vi "Get Number of Layers (SubVI).vi"(4 "error IN":errorcluster, 5 "Layers Array":T1(array[cluster]), 7 "VALUES clause IN":string) -> (0 "error OUT":errorcluster, 3 "VALUES clause OUT":string)   [LabVIEW 2010]
panel:
  out "numLayers":i32
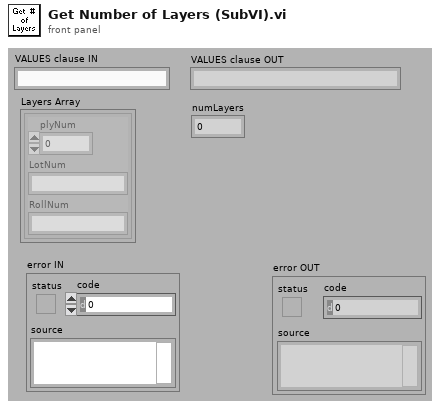
[diagram p1: front panel]
types:
  T1 = cluster{"plyNum":i32, "LotNum":string, "RollNum":string}[]
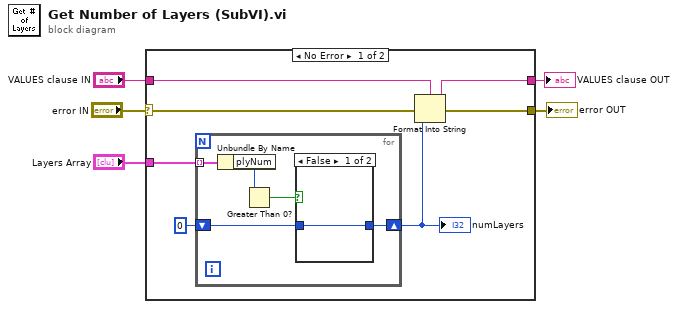
[diagram p0: block diagram]
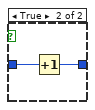
[diagram p2: hidden frame]
diagram:
  n1 = case shown="No Error" "error IN" {
    selector: "error IN" -> [w7 w21]
    tunnel: "Layers Array" -> [w11 _]
    tunnel: "VALUES clause IN" -> [w9 w22]
    tunnel: [w8 w22] -> w3
    tunnel: [w6 w21] -> w1
    frame No Error {
      n2 = for {
        tunnel: w11 -> [w15] mode=indexing
        shift-right: [w16] -> w10
        shift-left: 0 -> [w17]
        n3 = Unbundle By Name(w15) -> ("plyNum"=w14:i32)
        n4 = Greater Than 0?(x=w14) -> (x > 0?=w13:bool)
        n5 = case shown="False" w13 {
          tunnel: w17 -> [w18 w20]
          tunnel: [w18 w19] -> w16
          frame False {
          }
          frame True {
            n6 = Increment(x=w20) -> (x+1=w19:i32)
          }
        }
      }
      "numLayers" <- w10
      n7 = Format Into String(format string=w9, error in=w7, w10) -> (resulting string=w8:string, error out=w6:errorcluster)  [unwired: 1 in]
    }
    frame Error {
    }
  }
  "VALUES clause OUT" <- w3
  "error OUT" <- w1
